vi "Hold refnums open.vi"() -> ()   [LabVIEW 2012, in "Waveform Control.xctl"]
uses:
  Waveform Control.xctl
  Controls/Waveform State.ctl
  FP Controls.ctl
  Function Types.ctl
panel:
  in  "Name":string
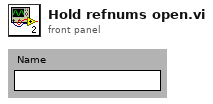
[diagram p1: front panel]
types:
  T1 = typedef "Waveform Control.xctl/Waveform State.ctl" = cluster{"Show Axes":bool, "Show Y=0":bool, "Controls":T2, "Show Current Location":bool, "Current Location":i32, "dt":dbl, "t0":timestamp, "Amplitude Format String":string}
  T2 = typedef "Waveform Control.xctl/FP Controls.ctl" = cluster{"Type":T3, "Periods":dbl, "Points":i32, "Offset":dbl, "Amplitdue":dbl, "Starting Phase":dbl, "func":string}
  T3 = typedef "Waveform Control.xctl/Function Types.ctl" = enum16{"Level", "Sine", "Triangle", "Ramp", "Saw Tooth", "Square", "Function"}
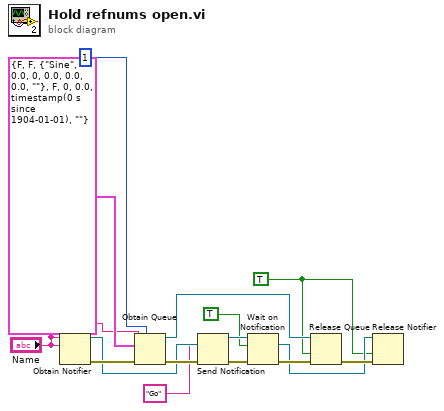
[diagram p0: block diagram]
diagram:
  w8 = TRUE ("force destroy? (F)")
  n1 = Obtain Notifier(name (unnamed)="Name", notification data type="Name") -> (notifier out=w6:refnum<notifier>, error out=w13:errorcluster)  [unwired: 2 in, 1 out]
  n2 = Obtain Queue(max queue size (-1, unlimited)=1, name (unnamed)="Name", element data type=T1 {"Show Axes"=FALSE, "Show Y=0"=FALSE, "Controls"={"Type"=enum."Sine", "Periods"=0.0, "Points"=0, "Offset"=0.0, "Amplitdue"=0.0, "Starting Phase"=0.0, "func"=""}, "Show Current Location"=FALSE, "Current Location"=0, "dt"=0.0, "t0"=timestamp(0 s since 1904-01-01), "Amplitude Format String"=""} ("State"), error in (no error)=w13) -> (queue out=w11:refnum<queue>, error out=w7:errorcluster)  [unwired: 1 in, 1 out]
  n3 = Send Notification(notification="Go", notifier=w6, error in (no error)=w7) -> (notifier out=w5:refnum<notifier>, error out=w4:errorcluster)
  n4 = Wait on Notification(notifier=w5, ignore previous (F)=TRUE, error in (no error)=w4) -> (notifier out=w9:refnum<notifier>, error out=w12:errorcluster)  [unwired: 3 out]
  n5 = Release Queue(queue=w11, force destroy? (F)=w8, error in (no error)=w12) -> (error out=w10:errorcluster)  [unwired: 2 out]
  n6 = Release Notifier(notifier=w9, force destroy? (F)=w8, error in (no error)=w10) -> ()  [unwired: 3 out]
